vi "Process.vi"(8 "error in (no error)":errorcluster, 10 "Pound in":refnum<class "Pound.lvclass">, 11 "Qbus in":refnum<class "Qbus.lvclass">) -> (0 "error out":errorcluster)   [LabVIEW 2017, in "EmsaTestPanel.lvlib"]
uses:
  <vilib>/addons/InsightCM/Devices/Shared/Emsa/EmsaTestPanel/EmsaTestPanel.lvlib
  <vilib>/addons/Qbus/Qbus.lvclass
  <vilib>/NI/Software Watchdog/Pound/Pound.lvclass
  <vilib>/addons/InsightCM/Devices/Shared/Emsa/EmsaTestPanel/controls/Configuration.ctl
  <vilib>/addons/InsightCM/Devices/Shared/Emsa/EmsaTestPanel/controls/DataSetType.ctl
  <vilib>/addons/InsightCM/Devices/Shared/Common/TestPanel/controls/Configuration.ctl
  <vilib>/addons/InsightCM/Devices/Shared/Common/TestPanel/controls/State.ctl
  <vilib>/addons/InsightCM/MessageBus/Base/controls/IRoutingSource.ctl
  <vilib>/addons/TraceLogger/TraceLogger.lvlib
  <vilib>/NI/Software Watchdog/Watchdog/Watchdog.lvclass
  <vilib>/addons/InsightCM/Devices/Shared/Common/DataFlow/DataFlow.lvlib
  <vilib>/addons/InsightCM/Utilities/GlobalConfiguration/GlobalConfiguration.lvlib
  <vilib>/addons/InsightCM/Devices/Shared/Common/ServerComm/ServerComm.lvlib
  <vilib>/addons/InsightCM/Devices/Shared/Common/TestPanel/TestPanel.lvlib
  <vilib>/addons/InsightCM/Devices/Shared/Emsa/EmsaAcquisition/EmsaAcquisition.lvlib
  <vilib>/addons/InsightCM/Devices/Shared/Emsa/EmsaAudio/EmsaAudio.lvlib
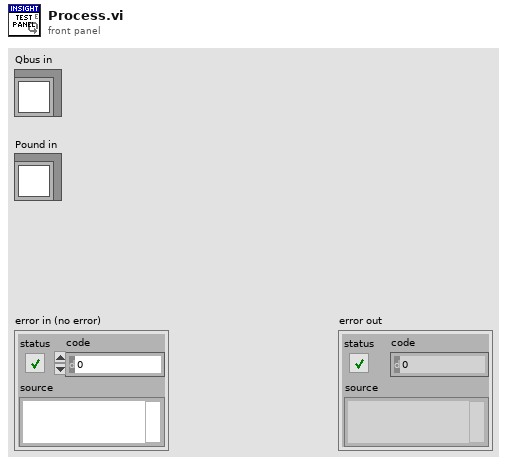
[diagram p1: front panel]
types:
  T1 = typedef "EmsaTestPanel.lvlib/Configuration.ctl" = cluster{"DataSet Type":T2, "ChanNameMap":variant, "Common":T3}
  T2 = typedef "EmsaTestPanel.lvlib/DataSetType.ctl" = enum16{"Waveform", "Sweep", "WAV"}
  T3 = typedef "TestPanel.lvlib/Configuration.ctl" = cluster{"State":T4, "Waveform Channel":string, "DataGroup":string, "Number of Samples":i32, "Waveform Length (sec)":dbl, "Timeout":dbl, "History":variant, "LastRequest":timestamp, "BufferSize":i32, "OpState":variant, "IRoutingSource":T5}
  T4 = typedef "TestPanel.lvlib/State.ctl" = enum16{"Off", "On", "PendingValues", "PendingDataSet"}
  T5 = typedef "IRoutingSource.ctl" = cluster{"CorrelationId":string, "ReplyTo":string}
  T6 = typedef "DataFlow.lvlib/Data.ctl" = cluster{"DataGroup":string, "Waveforms":T7, "Map":T8, "Type":T9}
  T7 = typedef "wfmSGL_DVR.ctl" = refnum<data-value>
  T8 = typedef "PointValueMap.lvlib/PointMap.ctl" = refnum<data-value>
  T9 = typedef "DataFlow.lvlib/Type.ctl" = enum16{"High Rate", "Low Rate", "Burst Mode"}
  T10 = typedef "EmsaAcquisition.lvlib/OnDemandWaveformData.ctl" = cluster{"Channel":string, "First Block":bool, "Last Block":bool, "Center Frequency":dbl, "Waveform":waveform(dbl)}
  T11 = typedef "EmsaAudio.lvlib/AudioFileCompleteBroadcast.ctl" = cluster{"Channel":string, "WAV file path":path}
  T12 = typedef "Message.ctl" = cluster{"Header":T13, "Body":u8[]}
  T13 = typedef "MessageHeader.ctl" = cluster{"MessageName":string, "Timestamp":i64, "CorrelationId":string, "ContentType":string, "RoutingKey":string, "Properties":T14[]}
  T14 = typedef "KeyValuePair.ctl" = cluster{"Key":string, "Value":string}
  T15 = typedef "DeviceTestPanelGetTimeSeriesRequestBody.ctl" = cluster{"DataGroup":string, "TrendPointIds":string[]}
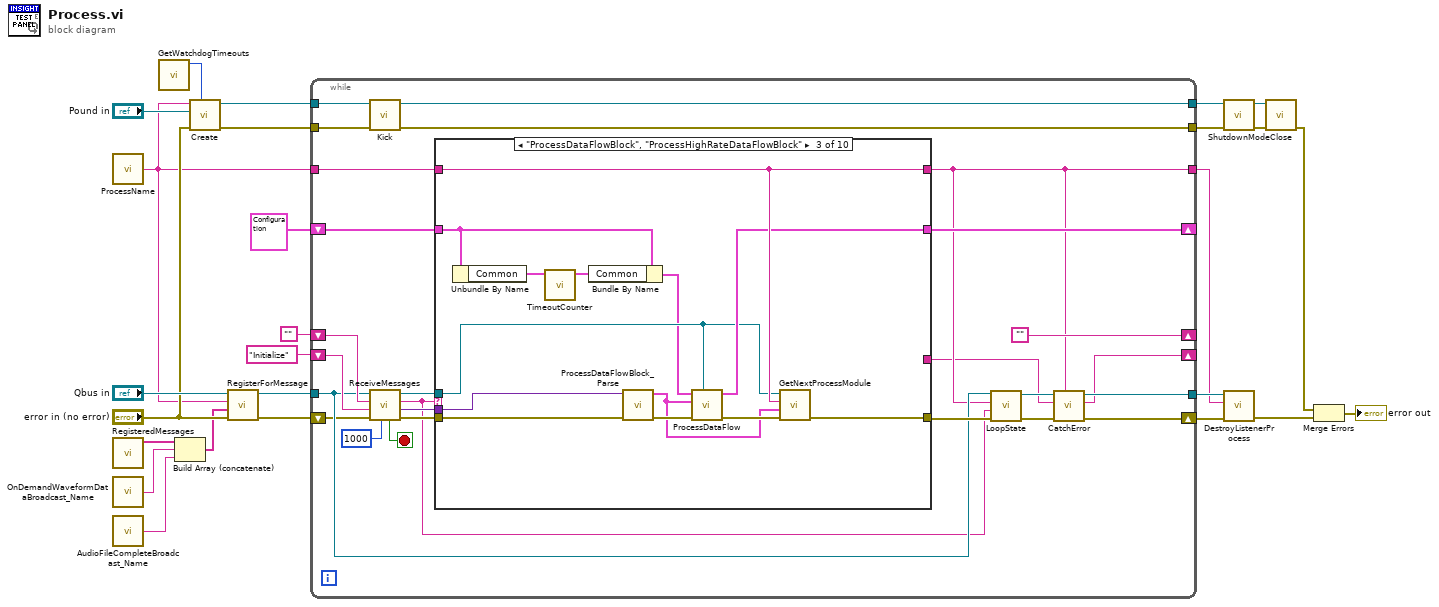
[diagram p0: block diagram]
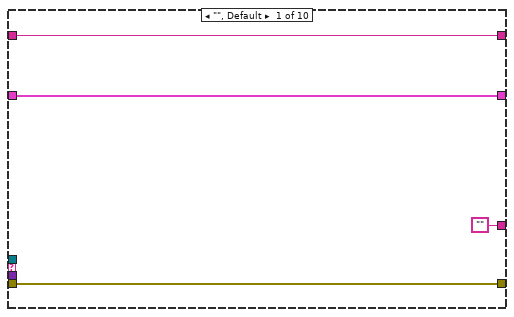
[diagram p2: hidden frame]
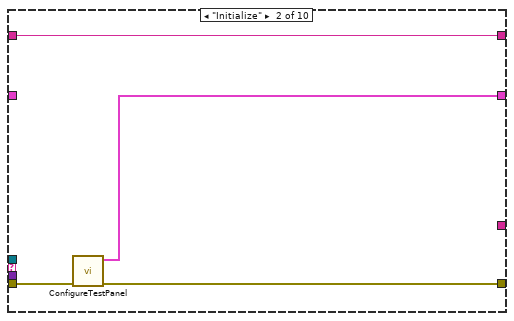
[diagram p3: hidden frame]
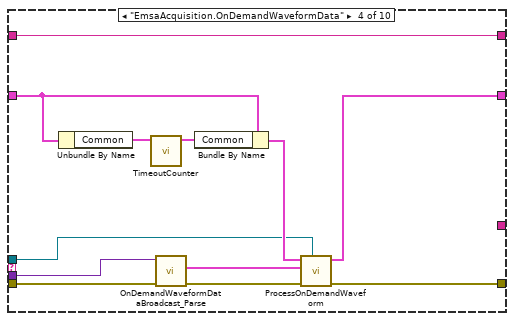
[diagram p4: hidden frame]
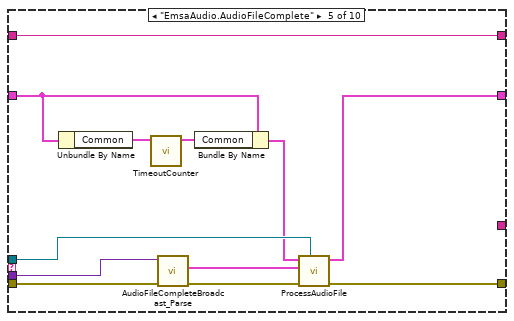
[diagram p5: hidden frame]
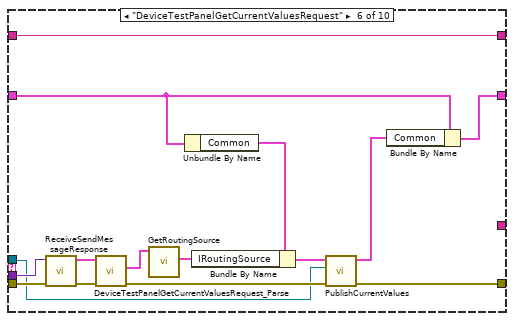
[diagram p6: hidden frame]
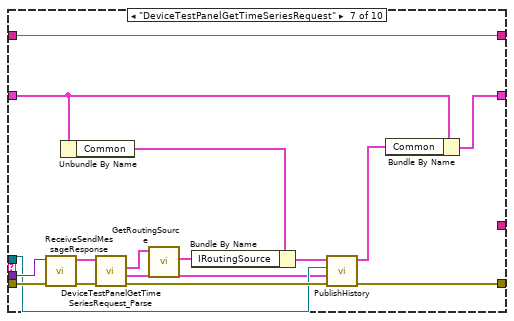
[diagram p7: hidden frame]
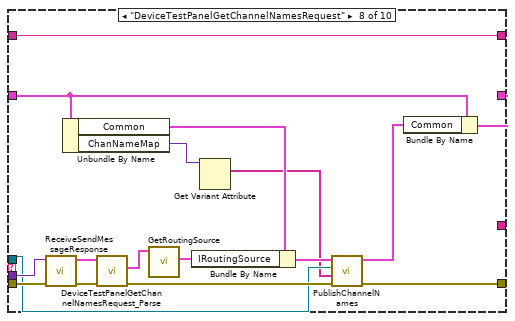
[diagram p8: hidden frame]
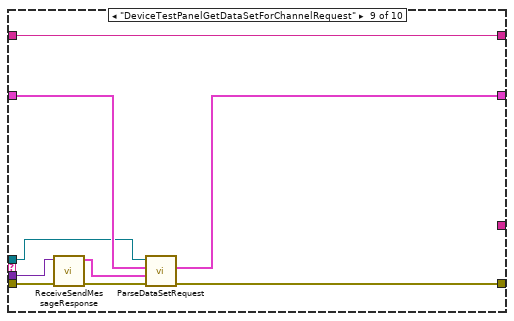
[diagram p9: hidden frame]
diagram:
  n1 = call <vilib>:"ProcessName.vi"() -> ("process name"=w6:string)  [unwired: 5 in]
  n2 = call <vilib>:"RegisteredMessages.vi"() -> ("registered messages"=w4:string[])  [unwired: 11 in]
  n3 = call <vilib>:"OnDemandWaveformDataBroadcast_Name.vi"() -> ("message name"=w2:string)  [unwired: 5 in]
  n4 = call <vilib>:"AudioFileCompleteBroadcast_Name.vi"() -> ("message name"=w1:string)  [unwired: 5 in]
  n5 = call <vilib>:"GetWatchdogTimeouts.vi"() -> ("software timeout"=w5:u32)  [unwired: 10 in, 1 out]
  n6 = Build Array (concatenate)(w4, w2, w1) -> (w3:string[])
  n7 = call <vilib>:"Create.vi"("Execution Timeout (ms)"=w5, "error in (no error)"="error in (no error)", "Pound"="Pound in", "Name"=w6) -> ("error out"=w15:errorcluster, "Watchdog"=w20:refnum<data-value>)  [unwired: 6 in]
  n8 = call <vilib>:"RegisterForMessage.vi"("error in (no error)"="error in (no error)", "message names"=w3, "process name"=w6, "Qbus in"="Qbus in") -> ("error in (no error)"=w7:errorcluster, "Qbus out"=w9:refnum<class "Qbus.lvclass">)  [unwired: 6 in]
  n9 = while {
    shift-right: [""] -> _
    shift-left: "" -> [w51]
    tunnel: w9 -> [w39]
    tunnel: w6 -> [w29]
    tunnel: [w42] -> w24
    tunnel: [w28] -> w23
    shift-right: [w41] -> _
    shift-left: "Initialize" -> [w46]
    shift-right: [w44] -> _
    shift-left: T1 {"DataSet Type"=enum."Waveform", "ChanNameMap"=variant, "Common"={"State"=enum."Off", "Waveform Channel"="", "DataGroup"="", "Number of Samples"=0, "Waveform Length (sec)"=0.0, "Timeout"=0.0, "History"=variant, "LastRequest"=timestamp(0 s since 1904-01-01), "BufferSize"=0, "OpState"=variant, "IRoutingSource"={"CorrelationId"="", "ReplyTo"=""}}} ("Test Panel Config") -> [w45]
    tunnel: w20 -> [w38]
    tunnel: [w37] -> w17
    tunnel: w15 -> [w36]
    tunnel: [w34] -> w14
    shift-right: [w43] -> w25
    shift-left: w7 -> [w35]
    stop <- w52 stop-if-true
    n10 = call <vilib>:"Kick.vi"("error in (no error)"=w36, "Watchdog"=w38) -> ("error out"=w34:errorcluster, "Watchdog"=w37:refnum<data-value>)  [unwired: 8 in]
    n11 = call <vilib>:"ReceiveMessages.vi"("Timeout(1000)"=1000 ("milliseconds to wait"), "error in (no error)"=w35, "priority action"=w46, "default action"=w51, "Qbus in"=w39) -> ("error out"=w50:errorcluster, "message value"=w47:variant, "action"=w33:string, "Qbus out"=w48:refnum<class "Qbus.lvclass">, "exit"=w52:bool)  [unwired: 2 in]
    n12 = case shown="\"ProcessDataFlowBlock\", \"ProcessHighRateDataFlowBlock\"" w33 {
      tunnel: w50 -> [w53 w60 w70 w80 w92 w111 w126 w143 w153 w157]
      tunnel: w48 -> [_ _ w65 w77 w91 w102 w114 w134 w147 _]
      tunnel: [w53 w57 w72 w75 w88 w101 w119 w135 w149 w157] -> w40
      tunnel: w47 -> [_ _ w71 w81 w93 w110 w123 w142 w152 _]
      tunnel: w45 -> [w56 _ w63 w83 w95 w100 w116 w132 w148 w156]
      tunnel: [w56 w59 w66 w76 w89 w99 w115 w131 w146 w156] -> w44
      tunnel: [w55 w58 w68 w85 w97 w112 w128 w145 w154 w155] -> w28
      tunnel: w29 -> [w55 w58 w68 w85 w97 w112 w128 w145 w154 w155]
      tunnel: ["" _ _ _ _ _ _ _ _ _] -> w27
      frame "", Default {
      }
      frame "Initialize" {
        n13 = call <vilib>:"ConfigureTestPanel.vi"("error in (no error)"=w60) -> ("error out"=w57:errorcluster, "Test Panel Config out"=w59:T1)  [unwired: 9 in]
      }
      frame "ProcessDataFlowBlock", "ProcessHighRateDataFlowBlock" {
        n14 = Unbundle By Name(w63) -> ("Common"=w64:T3)
        n15 = call <vilib>:"TimeoutCounter.vi"("config in"=w64) -> ("config out"=w62:T3)  [unwired: 10 in]
        n16 = Bundle By Name(cluster=w63, "Common"=w62) -> (w61:T1)
        n17 = call <vilib>:"ProcessDataFlowBlock_Parse.vi"("error in (no error)"=w70, "body"=w71) -> ("error out"=w69:errorcluster, "data"=w67:T6)  [unwired: 8 in]
        n18 = call <vilib>:"ProcessDataFlow.vi"("Qbus in"=w65, "error in (no error)"=w69, "Data"=w67, "config in"=w61) -> ("error out"=w73:errorcluster, "config out"=w66:T1)  [unwired: 6 in]
        n19 = call <vilib>:"GetNextProcessModule.vi"("error in (no error)"=w73, "data"=w67, "source"=w68, "Qbus in"=w65) -> ("error out"=w72:errorcluster)  [unwired: 6 in, 1 out]
      }
      frame "EmsaAcquisition.OnDemandWaveformData" {
        n20 = Unbundle By Name(w83) -> ("Common"=w84:T3)
        n21 = call <vilib>:"TimeoutCounter.vi"("config in"=w84) -> ("config out"=w82:T3)  [unwired: 10 in]
        n22 = call <vilib>:"OnDemandWaveformDataBroadcast_Parse.vi"("error in (no error)"=w80, "message"=w81) -> ("error out"=w79:errorcluster, "on demand waveform"=w74:T10)  [unwired: 8 in]
        n23 = Bundle By Name(cluster=w83, "Common"=w82) -> (w78:T1)
        n24 = call <vilib>:"ProcessOnDemandWaveform.vi"("Qbus in"=w77, "error in (no error)"=w79, "on demand waveform"=w74, "config in"=w78) -> ("error out"=w75:errorcluster, "config out"=w76:T1)  [unwired: 6 in]
      }
      frame "EmsaAudio.AudioFileComplete" {
        n25 = Unbundle By Name(w95) -> ("Common"=w96:T3)
        n26 = call <vilib>:"TimeoutCounter.vi"("config in"=w96) -> ("config out"=w94:T3)  [unwired: 10 in]
        n27 = call <vilib>:"AudioFileCompleteBroadcast_Parse.vi"("error in (no error)"=w92, "message"=w93) -> ("error out"=w87:errorcluster, "data"=w86:T11)  [unwired: 8 in]
        n28 = Bundle By Name(cluster=w95, "Common"=w94) -> (w90:T1)
        n29 = call <vilib>:"ProcessAudioFile.vi"("Qbus in"=w91, "error in (no error)"=w87, "data"=w86, "config in"=w90) -> ("error out"=w88:errorcluster, "config out"=w89:T1)  [unwired: 6 in]
      }
      frame "DeviceTestPanelGetCurrentValuesRequest" {
        n30 = call <vilib>:"ReceiveSendMessageResponse.vi"("error in (no error)"=w111, "body"=w110) -> ("error out"=w109:errorcluster, "message"=w108:T12)  [unwired: 6 in, 2 out]
        n31 = call <vilib>:"DeviceTestPanelGetCurrentValuesRequest_Parse.vi"("error in (no error)"=w109, "Message"=w108) -> ("error out"=w103:errorcluster, "Header"=w107:T13)  [unwired: 7 in, 1 out]
        n32 = call <vilib>:"GetRoutingSource.vi"("Header in"=w107) -> ("IRoutingSource"=w106:T5)  [unwired: 9 in, 1 out]
        n33 = Unbundle By Name(w100) -> ("Common"=w105:T3)
        n34 = Bundle By Name(cluster=w105, "IRoutingSource"=w106) -> (w104:T3)
        n35 = call <vilib>:"PublishCurrentValues.vi"("error in (no error)"=w103, "Qbus in"=w102, "config in"=w104) -> ("error out"=w101:errorcluster, "config out"=w98:T3)  [unwired: 7 in]
        n36 = Bundle By Name(cluster=w100, "Common"=w98) -> (w99:T1)
      }
      frame "DeviceTestPanelGetTimeSeriesRequest" {
        n37 = call <vilib>:"ReceiveSendMessageResponse.vi"("error in (no error)"=w126, "body"=w123) -> ("error out"=w125:errorcluster, "message"=w124:T12)  [unwired: 6 in, 2 out]
        n38 = Unbundle By Name(w116) -> ("Common"=w121:T3)
        n39 = call <vilib>:"DeviceTestPanelGetTimeSeriesRequest_Parse.vi"("error in (no error)"=w125, "Message"=w124) -> ("error out"=w120:errorcluster, "Body"=w113:T15, "Header"=w122:T13)  [unwired: 6 in, 1 out]
        n40 = call <vilib>:"GetRoutingSource.vi"("Header in"=w122) -> ("IRoutingSource"=w127:T5)  [unwired: 9 in, 1 out]
        n41 = Bundle By Name(cluster=w121, "IRoutingSource"=w127) -> (w118:T3)
        n42 = call <vilib>:"PublishHistory.vi"("error in (no error)"=w120, "Body"=w113, "Qbus in"=w114, "config in"=w118) -> ("error out"=w119:errorcluster, "config out"=w117:T3)  [unwired: 6 in]
        n43 = Bundle By Name(cluster=w116, "Common"=w117) -> (w115:T1)
      }
      frame "DeviceTestPanelGetChannelNamesRequest" {
        n44 = call <vilib>:"ReceiveSendMessageResponse.vi"("error in (no error)"=w143, "body"=w142) -> ("error out"=w140:errorcluster, "message"=w141:T12)  [unwired: 6 in, 2 out]
        n45 = Unbundle By Name(w132) -> ("Common"=w138:T3, "ChanNameMap"=w130:variant)
        n46 = call <vilib>:"DeviceTestPanelGetChannelNamesRequest_Parse.vi"("error in (no error)"=w140, "Message"=w141) -> ("error out"=w136:errorcluster, "Header"=w139:T13)  [unwired: 7 in, 1 out]
        n47 = call <vilib>:"GetRoutingSource.vi"("Header in"=w139) -> ("IRoutingSource"=w144:T5)  [unwired: 9 in, 1 out]
        n48 = Bundle By Name(cluster=w138, "IRoutingSource"=w144) -> (w137:T3)
        n49 = Get Variant Attribute(Variant=w130) -> (names=w129:string[])  [unwired: 3 in, 3 out]
        n50 = call <vilib>:"PublishChannelNames.vi"("error in (no error)"=w136, "names"=w129, "Qbus in"=w134, "config in"=w137) -> ("error out"=w135:errorcluster, "config out"=w133:T3)  [unwired: 6 in]
        n51 = Bundle By Name(cluster=w132, "Common"=w133) -> (w131:T1)
      }
      frame "DeviceTestPanelGetDataSetForChannelRequest" {
        n52 = call <vilib>:"ReceiveSendMessageResponse.vi"("error in (no error)"=w153, "body"=w152) -> ("error out"=w150:errorcluster, "message"=w151:T12)  [unwired: 6 in, 2 out]
        n53 = call <vilib>:"ParseDataSetRequest.vi"("error in (no error)"=w150, "message"=w151, "config"=w148, "Qbus in"=w147) -> ("error out"=w149:errorcluster, "config out"=w146:T1)  [unwired: 6 in]
      }
      frame "Exit" {
      }
    }
    n54 = call <vilib>:"LoopState.vi"("error in (no error)"=w40, "loop action"=w33, "process name"=w28, "Qbus in"=w39) -> ("error out"=w31:errorcluster, "Qbus out"=w30:refnum<class "Qbus.lvclass">)  [unwired: 6 in]
    n55 = call <vilib>:"CatchError.vi"("source"=w28, "error in (no error)"=w31, "next action in"=w27, "Qbus in"=w30) -> ("error out"=w43:errorcluster, "next action out"=w41:string, "Qbus out"=w42:refnum<class "Qbus.lvclass">)  [unwired: 5 in]
  }
  n56 = call <vilib>:"ShutdownMode.vi"("error in (no error)"=w14, "Watchdog"=w17) -> ("error out"=w16:errorcluster, "Watchdog"=w18:refnum<data-value>)  [unwired: 8 in]
  n57 = call <vilib>:"DestroyListenerProcess.vi"("error in (no error)"=w25, "process name"=w23, "Qbus in"=w24) -> ("error in (no error)"=w13:errorcluster)  [unwired: 7 in, 1 out]
  n58 = call <vilib>:"Close.vi"("error in (no error)"=w16, "Watchdog"=w18) -> ("error out"=w12:errorcluster)  [unwired: 9 in]
  n59 = Merge Errors(w12, w13) -> (→"error out":errorcluster)
